vi "worksheet outline settings.vi"(6 "auto_style":u8, 7 "symbols_right":u8, 8 "error in (no error)":errorcluster, 9 "symbols_below":u8, 10 "visible":u8, 11 "worksheet":u32) -> (0 "error out":errorcluster)   [LabVIEW 8.6]
doc: "void worksheet_outline_settings(lxw_worksheet worksheet, uint8_t visible, uint8_t symbols_below, uint8_t symbols_right, uint8_t auto_style);"
uses:
  pending_lvxlsxwriter/xlsxwriter.dll
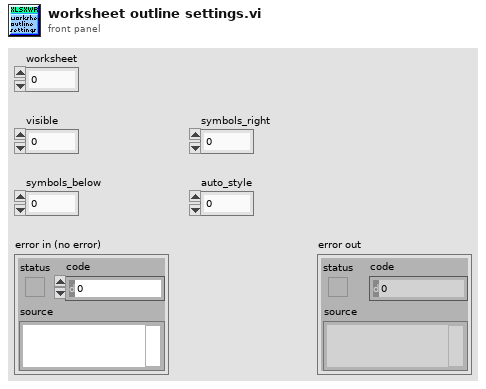
[diagram p1: front panel]
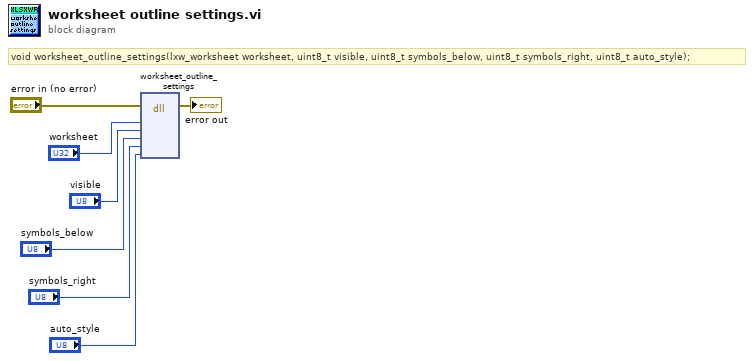
[diagram p0: block diagram]
diagram:
  # "void worksheet_outline_settings(lxw_worksheet worksheet, uint8_t visible, uint8_t symbols_below, uint8_t symbols_right, uint8_t auto_style);"
  n1 = dll-call lib="C:/Users/WDAGUtilityAccount/Desktop/pending_lvxlsxwriter/xlsxwriter.*" fn="worksheet_outline_settings"(error in="error in (no error)", "worksheet"="worksheet", "visible"="visible", "symbols_below"="symbols_below", "symbols_right"="symbols_right", "auto_style"="auto_style") -> (error out=→"error out":errorcluster)  [unwired: 8 in, 1 out]
